vi "3D Curve Graph (ActiveX).vi"() -> ()   [LabVIEW 2023]
doc: "This VI illustrates the use of 3D Curves to display the numerical solution of the Lorentz dynamical model of convection phenomena used in meteorological systems.\n\nWith the default values, it creates a chaotic attractor in three dimensions, using the basic Lorenz equations (i.e without Forcing Functions). The parameters of the Lorentz model can be modified to illustrate different types of behavioral response of the system.\n\nThe largest performance disadvantage for the 3D graph is rendering the data to the screen, and this example demonstrates the efficiency of computing an entire data set before displaying it."
uses:
  <vilib>/Platform/NI_3dgraph.lvlib
panel:
  in  "3D Curve - Lorenz Attractor":refnum<k7>(container)
  # "Overview: Demonstrates the ActiveX 3D Curve Graph.vi control.\nRequirements: Windows\nInstructions:\nRun the VI. The solution to a Lorenz equation is displayed in the graph. See the block diagram for more information."
  # "The ActiveX 3D Curve Graph.vi is located in the Classic > Classic Graph palette."
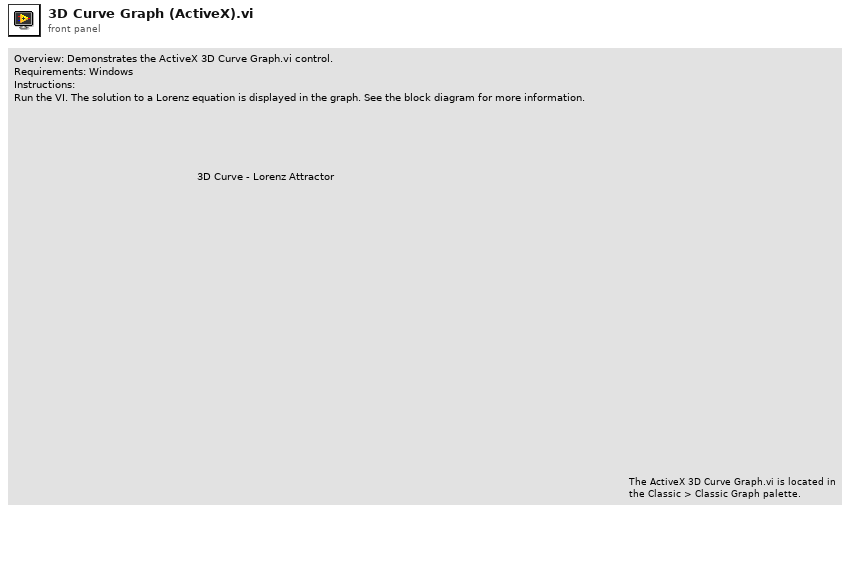
[diagram p1: front panel]
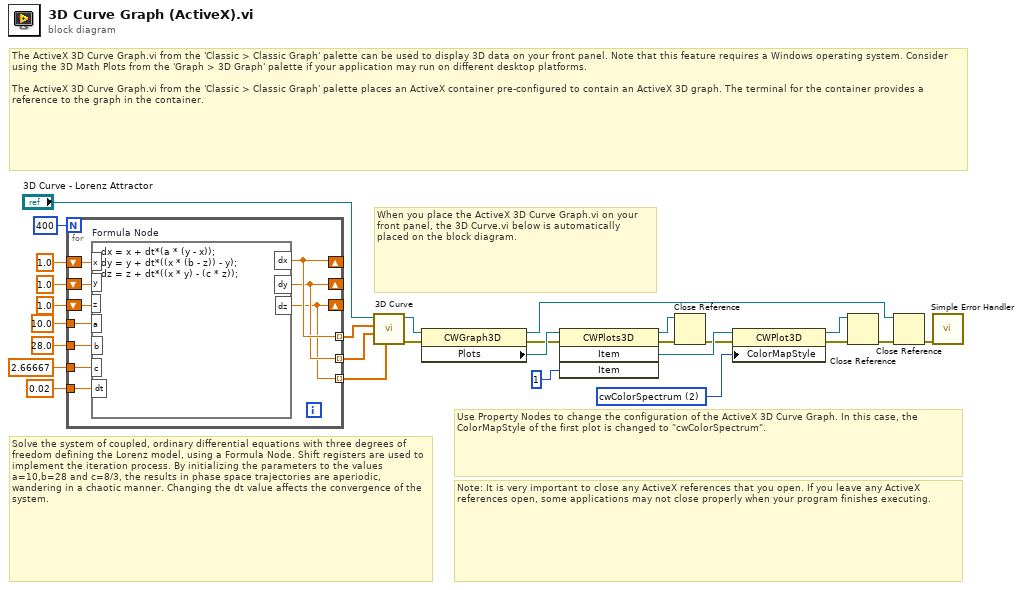
[diagram p0: block diagram]
diagram:
  w14 = 2 items=["cwNone", "cwShaded", "cwColorSpectrum", "cwGrayScale"] ("ColorMapStyle")
  # "When you place the ActiveX 3D Curve Graph.vi on your front panel, the 3D Curve.vi below is automatically placed on the block diagram."
  # "The ActiveX 3D Curve Graph.vi from the 'Classic > Classic Graph' palette can be used to display 3D data on your front panel. Note that this feature requires a Windows operating system. Consider using the 3D Math Plots from the 'Graph > 3D Graph' palette if your application may run on different desktop platforms.\n\nThe ActiveX 3D Curve Graph.vi from the 'Classic > Classic Graph' palette places an ActiveX container pre-configured to contain an ActiveX 3D graph. The terminal for the container provides a reference to the graph in the container."
  # "Note: It is very important to close any ActiveX references that you open. If you leave any ActiveX references open, some applications may not close properly when your program finishes executing."
  # "Use Property Nodes to change the configuration of the ActiveX 3D Curve Graph. In this case, the ColorMapStyle of the first plot is changed to \"cwColorSpectrum\"."
  # "Solve the system of coupled, ordinary differential equations with three degrees of freedom defining the Lorenz model, using a Formula Node. Shift registers are used to implement the iteration process. By initializing the parameters to the values a=10,b=28 and c=8/3, the results in phase space trajectories are aperiodic, wandering in a chaotic manner. Changing the dt value affects the convergence of the system."
  n1 = for {
    N: 400 -> [_]
    tunnel: 0.02 ("dt") -> [w28]
    tunnel: [w29] -> w17 mode=indexing
    tunnel: [w30] -> w18 mode=indexing
    tunnel: [w31] -> w19 mode=indexing
    shift-left: 1.0 ("Z") -> [w32]
    shift-right: [w29] -> _
    shift-left: 1.0 ("Y") -> [w33]
    shift-right: [w30] -> _
    shift-left: 1.0 ("X") -> [w34]
    shift-right: [w31] -> _
    tunnel: 2.66667 ("c") -> [w35]
    tunnel: 28.0 ("b") -> [w36]
    tunnel: 10.0 ("a") -> [w37]
    n2 = formula code="dx = x + dt*(a * (y - x));\ndy = y + dt*((x * (b - z)) - y);\ndz = z + dt*((x * y) - (c * z));"("x"=w34, "y"=w33, "z"=w32, "a"=w37, "b"=w36, "c"=w35, "dt"=w28) -> ("dx"=w31:dbl, "dy"=w30:dbl, "dz"=w29:dbl)
  }
  n3 = call <vilib>:"3D Curve.vi"("z vector"=w17, "y vector"=w18, "x vector"=w19, "3D graph"="3D Curve - Lorenz Attractor") -> ("error out"=w12:errorcluster, "3D graph out"=w11:refnum<k7>)  [unwired: 6 in]
  n4 = property class="CWGraph3D"(reference=w11, error in=w12) -> (reference out=w2:refnum<k7>, error out=w10:errorcluster, "Plots"=w15:refnum<k7>)
  n5 = invoke class="CWPlots3D" method="Item"(reference=w15, error in=w10, "Item"=1) -> (reference out=w8:refnum<k7>, error out=w9:errorcluster, "Item"=w13:refnum<k7>)  [unwired: 1 in, 1 out]
  n6 = Close Reference(reference=w8, error in (no error)=w9) -> (error out=w7:errorcluster)
  n7 = property class="CWPlot3D"(reference=w13, error in=w7, "ColorMapStyle"=w14) -> (reference out=w5:refnum<k7>, error out=w6:errorcluster)
  n8 = Close Reference(reference=w5, error in (no error)=w6) -> (error out=w3:errorcluster)
  n9 = Close Reference(reference=w2, error in (no error)=w3) -> (error out=w4:errorcluster)
  n10 = call <vilib>:"Simple Error Handler.vi"("error in (no error)"=w4) -> ()  [unwired: 4 in, 5 out]
